vi "SDCP - Serial Port Control Test.vi"() -> ()   [LabVIEW 2020]
uses:
  Typedefs/SDCP - Serial Port Control - Commands.ctl
panel:
  out "Rx Log time":u32[](array[numeric])
  out "Rx Log":string[](array[string])
  out "Update Rx table":bool
  in  "Receive table":i32(listbox)
  in  "Transmit table":i32(listbox)
  in  "Bytes to transmit":u8[](array[numeric])
  in  "Transmit bytes":bool
  out "Received bytes":u8[](array[numeric])
  in  "Number of bytes to read":u32
  out "Stop Application Flag":bool
  in  "Stop Application":bool
  out "Connected":bool
  in  "Serial Port Connect/Disconnect":bool
  in  "COM Port":refnum<visa-resource-name>
  in  "Baud rate":u32=9600
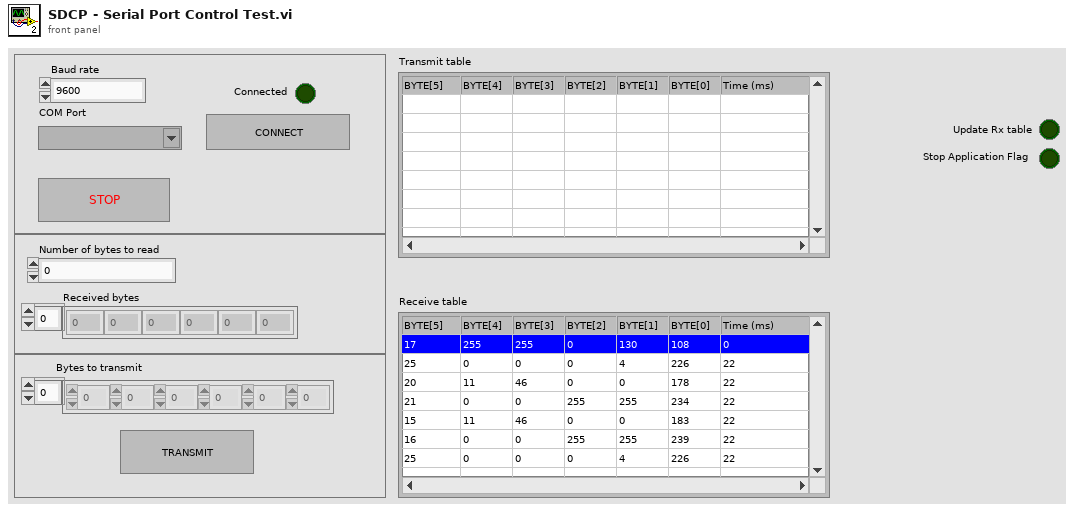
[diagram p1: front panel]
types:
  T1 = typedef "SDCP - Serial Port Control - Commands.ctl" = enum16{"Open", "Read", "Write", "Get instance", "Close"}
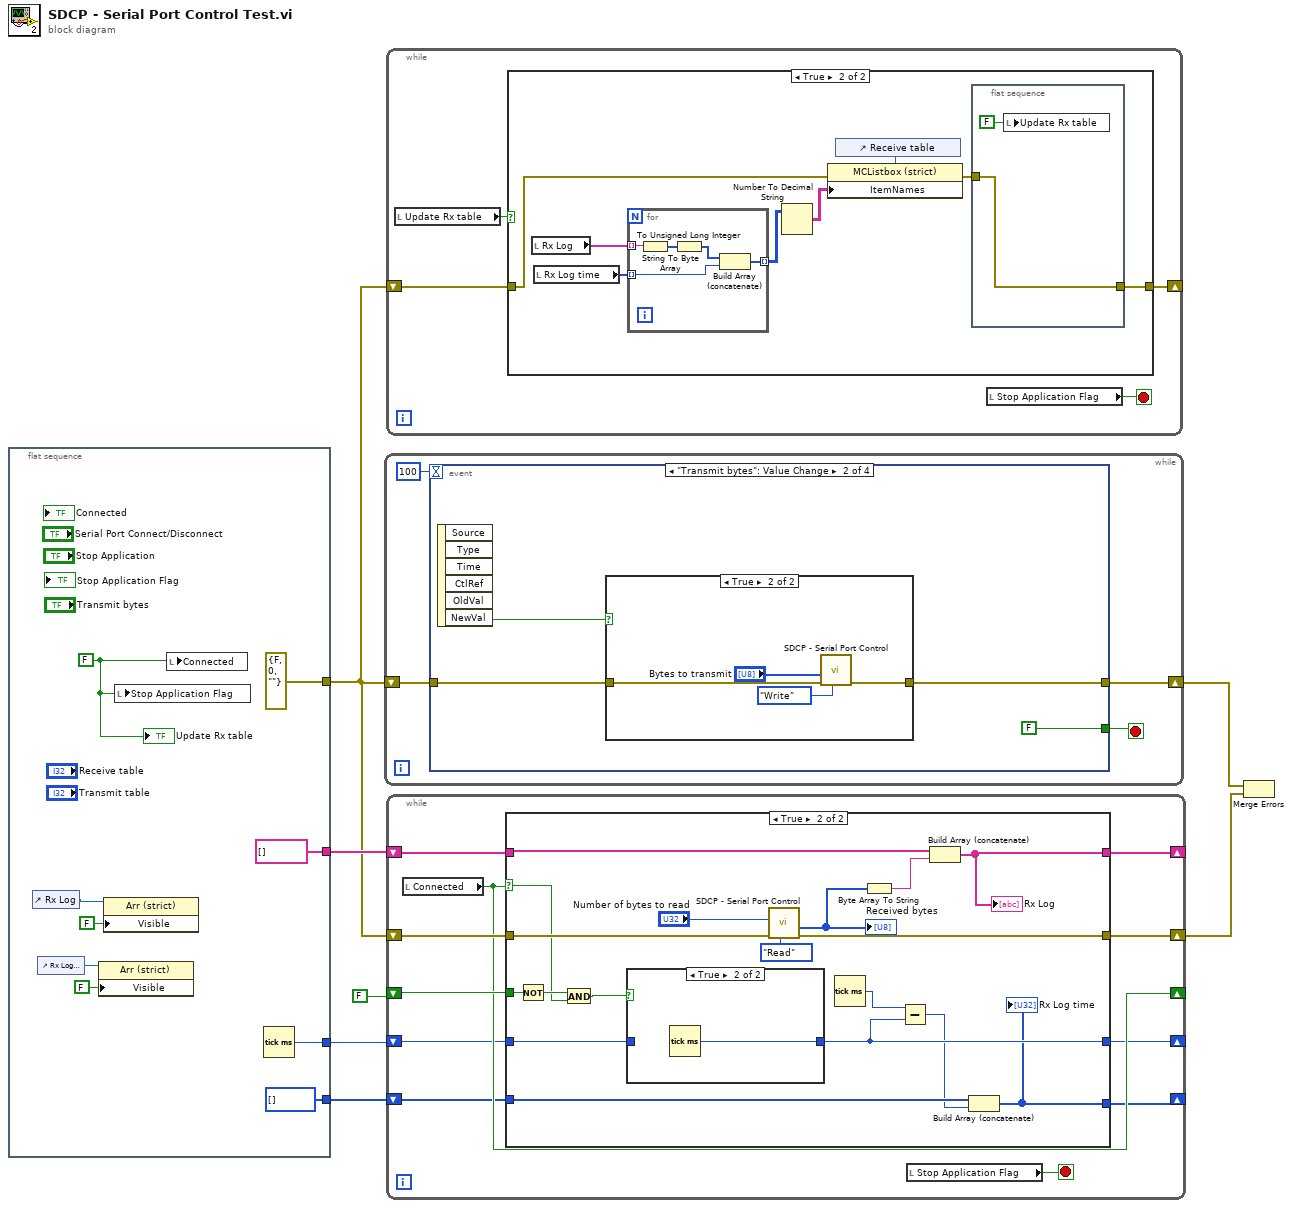
[diagram p0: block diagram]
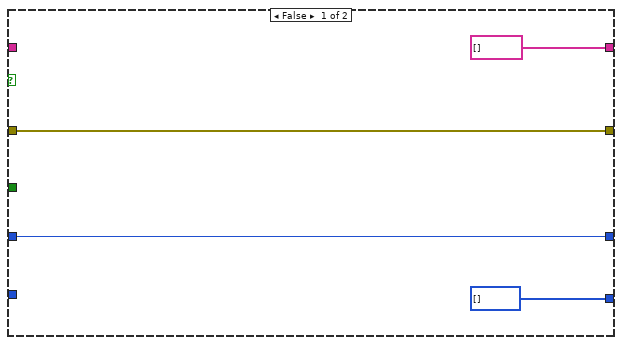
[diagram p3: hidden frame]
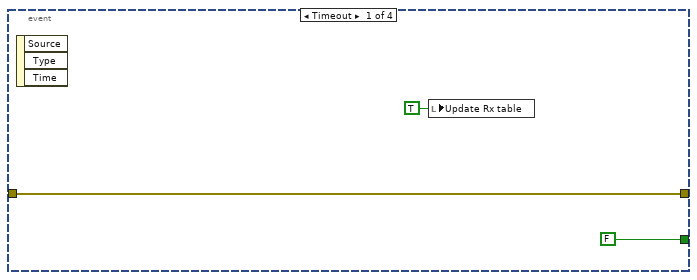
[diagram p5: hidden frame]
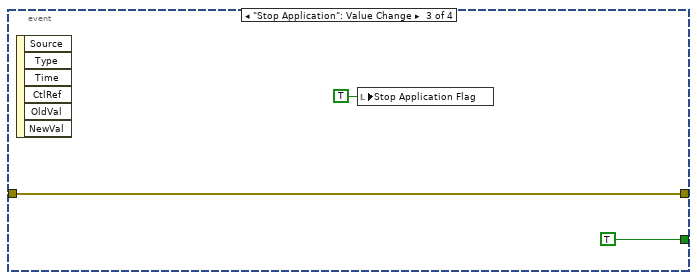
[diagram p7: hidden frame]
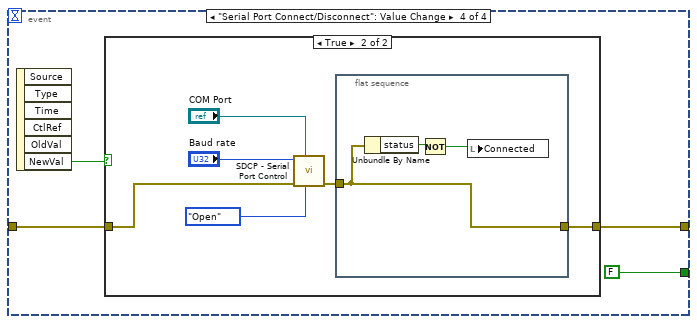
[diagram p8: hidden frame]
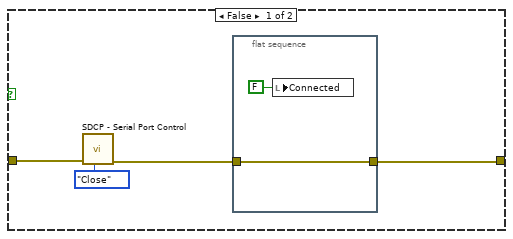
[diagram p9: hidden frame]
diagram:
  n1 = flat-sequence {
    tunnel: [errorcluster {"status"=FALSE, "code"=0, "source"=""} ("error constant")] -> w1
    tunnel: [string[] []] -> w5
    tunnel: [w14] -> w3
    tunnel: [i32[] []] -> w2
    frame #0 {
      w12 = FALSE
      n2 = control-ref of="Rx Log"() -> (w11:refnum<vi>)
      n3 = control-ref of="Rx Log time"() -> (w9:refnum<vi>)
      n4 = property class="Arr (strict)"(reference=w9, "Visible"=FALSE) -> ()  [unwired: 1 in, 2 out]
      n5 = property class="Arr (strict)"(reference=w11, "Visible"=FALSE) -> ()  [unwired: 1 in, 2 out]
      n6 = local write "Stop Application Flag"(w12) -> ()
      n7 = local write "Connected"(w12) -> ()
      n8 = Tick Count (ms)() -> (millisecond timer value=w14:u32)
      "Update Rx table" <- w12
    }
  }
  n9 = while {
    shift-right: [w20] -> w7
    shift-left: w1 -> [w19]
    stop <- w18 stop-if-true
    n10 = event shown="[1] \"Transmit bytes\": Value Change" {
      selector: _ -> [_ _ _ _]
      dyn-events: _ -> [_ _ _ _]
      timeout: 100 -> [_ _ _ _]
      tunnel: [w23 w26 w35 w38] -> w20
      tunnel: w19 -> [w23 w27 w35 w37]
      tunnel: [FALSE FALSE TRUE FALSE] -> w18
      event Timeout {
        n11 = event-data() -> ()  [unwired: 1 in, 3 out]
        n12 = local write "Update Rx table"(TRUE ("Update Rx table")) -> ()
      }
      event "Transmit bytes": Value Change {
        n13 = event-data() -> ("NewVal"=w24:bool)  [unwired: 1 in, 5 out]
        n14 = case shown="True" w24 {
          tunnel: w27 -> [w28 w32]
          tunnel: [w28 w29] -> w26
          frame False {
          }
          frame True {
            n15 = call "SDCP - Serial Port Control.vi"("Command"=SDCP_-_Serial_Port_Control_-_Commands."Write", "error in (no error)"=w32, "Transmit bytes"="Bytes to transmit") -> ("error out"=w29:errorcluster)  [unwired: 7 in, 1 out]
          }
        }
      }
      event "Stop Application": Value Change {
        n16 = event-data() -> ()  [unwired: 1 in, 6 out]
        n17 = local write "Stop Application Flag"(TRUE ("Stop Application Flag")) -> ()
      }
      event "Serial Port Connect/Disconnect": Value Change {
        n18 = event-data() -> ("NewVal"=w39:bool)  [unwired: 1 in, 5 out]
        n19 = case shown="True" w39 {
          tunnel: [w40 w46] -> w38
          tunnel: w37 -> [w42 w48]
          frame False {
            n20 = call "SDCP - Serial Port Control.vi"("Command"=SDCP_-_Serial_Port_Control_-_Commands."Close", "error in (no error)"=w42) -> ("error out"=w41:errorcluster)  [unwired: 8 in, 1 out]
            n21 = flat-sequence {
              tunnel: w41 -> [w44]
              tunnel: [w44] -> w40
              frame #0 {
                n22 = local write "Connected"(FALSE ("Connected")) -> ()
              }
            }
          }
          frame True {
            n23 = call "SDCP - Serial Port Control.vi"("Command"=SDCP_-_Serial_Port_Control_-_Commands."Open", "VISA resource name"="COM Port", "error in (no error)"=w48, "Baud rate"="Baud rate") -> ("error out"=w47:errorcluster)  [unwired: 6 in, 1 out]
            n24 = flat-sequence {
              tunnel: w47 -> [w54]
              tunnel: [w54] -> w46
              frame #0 {
                n25 = Unbundle By Name(w54) -> ("status"=w53:bool)
                n26 = Not(x=w53) -> (.not. x?=w52:bool)
                n27 = local write "Connected"(w52) -> ()
              }
            }
          }
        }
      }
    }
  }
  n28 = while {
    shift-right: [w55] -> _
    shift-left: w1 -> [w56]
    stop <- w58 stop-if-true
    n29 = local read "Update Rx table"() -> (w57:bool)
    n30 = case shown="True" w57 {
      tunnel: w56 -> [w59 w66]
      tunnel: [w59 w60] -> w55
      frame False {
      }
      frame True {
        n31 = local read "Rx Log"() -> (w65:string[])
        n32 = local read "Rx Log time"() -> (w64:u32[])
        n33 = for {
          tunnel: w65 -> [w74] mode=indexing
          tunnel: w64 -> [w72] mode=indexing
          tunnel: [w70] -> w63 mode=indexing
          n34 = String To Byte Array(string=w74) -> (unsigned byte array=w73:u8[])
          n35 = To Unsigned Long Integer(number=w73) -> (unsigned 32bit integer=w71:u32[])
          n36 = Build Array (concatenate)(w71, w72) -> (w70:u32[])
        }
        n37 = Number To Decimal String(number=w63) -> (decimal integer string=w62:string[][])  [unwired: 1 in]
        n38 = control-ref of="Receive table"() -> (w67:refnum<vi>)
        n39 = property class="MCListbox (strict)"(reference=w67, error in=w66, "ItemNames"=w62) -> (error out=w61:errorcluster)  [unwired: 1 out]
        n40 = flat-sequence {
          tunnel: w61 -> [w69]
          tunnel: [w69] -> w60
          frame #0 {
            n41 = local write "Update Rx table"(FALSE ("Update Rx table")) -> ()
          }
        }
      }
    }
    n42 = local read "Stop Application Flag"() -> (w58:bool)
  }
  n43 = while {
    shift-right: [w83] -> w6
    shift-left: w1 -> [w84]
    shift-right: [w81] -> _
    shift-left: w5 -> [w82]
    shift-right: [w79] -> _
    shift-left: FALSE -> [w80]
    shift-right: [w77] -> _
    shift-left: w3 -> [w78]
    shift-right: [w75] -> _
    shift-left: w2 -> [w76]
    stop <- w85 stop-if-true
    n44 = local read "Connected"() -> (w79:bool)
    n45 = case shown="True" w79 {
      selector: w79 -> [_ w97]
      tunnel: w84 -> [w89 w107]
      tunnel: [w89 w104] -> w83
      tunnel: w82 -> [_ w102]
      tunnel: [string[] [] w101] -> w81
      tunnel: w80 -> [_ w98]
      tunnel: w78 -> [w88 w95]
      tunnel: [w88 w94] -> w77
      tunnel: w76 -> [_ w92]
      tunnel: [u32[] [] w91] -> w75
      frame False {
      }
      frame True {
        n46 = Not(x=w98) -> (.not. x?=w99:bool)
        n47 = And(x=w99, y=w97) -> (x .and. y?=w96:bool)
        n48 = case shown="True" w96 {
          tunnel: [w108 w109] -> w94
          tunnel: w95 -> [w108 _]
          frame False {
          }
          frame True {
            n49 = Tick Count (ms)() -> (millisecond timer value=w109:u32)
          }
        }
        n50 = call "SDCP - Serial Port Control.vi"("Command"=SDCP_-_Serial_Port_Control_-_Commands."Read", "error in (no error)"=w107, "Read byte count"="Number of bytes to read") -> ("error out"=w104:errorcluster, "Received bytes"=w103:u8[])  [unwired: 7 in]
        "Received bytes" <- w103
        n51 = Tick Count (ms)() -> (millisecond timer value=w93:u32)
        n52 = Byte Array To String(unsigned byte array=w103) -> (string=w100:string)
        n53 = Subtract(x=w93, y=w94) -> (x-y=w90:u32)
        n54 = Build Array (concatenate)(w102, w100) -> (w101:string[])
        "Rx Log" <- w101
        n55 = Build Array (concatenate)(w92, w90) -> (w91:u32[])
        "Rx Log time" <- w91
      }
    }
    n56 = local read "Stop Application Flag"() -> (w85:bool)
  }
  n57 = Merge Errors(w7, w6) -> ()  [unwired: 1 out]
